vi "Read All Devices States.vi"(8 "error in (no error)":errorcluster, 11 "Data Cluster":T1 {"Flexi-Flow Devices"."Control State"."Control Mode" items=["Bus/RS232"=0, "FLOW-BUS slave"=2, "Valve close"=3, "Controller idle"=4, "Setpoint 100%"=7, "Valve fully open"=8, "Calibration mode"=9, "Setpoint 0%"=12, "RS232"=18, "Valve steering"=20, "Valve safe state"=22]}) -> (0 "error out":errorcluster, 1 "Array":sgl[](array[numeric]), 2 "Data Table":map{string, dbl}(c390), 3 "Array Out":T3[](array[typedef]) {"Control State"."Control Mode" items=["Bus/RS232"=0, "FLOW-BUS slave"=2, "Valve close"=3, "Controller idle"=4, "Setpoint 100%"=7, "Valve fully open"=8, "Calibration mode"=9, "Setpoint 0%"=12, "RS232"=18, "Valve steering"=20, "Valve safe state"=22]})   [LabVIEW 2024, in "FlexiFlowInterfaceCH2.lvlib"]
uses:
  FlexiFlowInterfaceCH2.lvlib
  Modbus Flexi-Flow State--cluster.ctl
  <vilib>/Plasmionique/MB Master/MB_Master_TCP/MB_Master_TCP.lvclass
  Device Type--enum.ctl
  Modbus Flexi-Flow Controls--cluster.ctl
  Modbus Flexi-Flow API/Control Mode--enum.ctl
  Modbus Flexi-Flow API/Control Function Values--enum.ctl
  Modbus Flexi-Flow Measure State--cluster.ctl
  Module Data--cluster.ctl
  Modbus TCP Connection Settings--cluster.ctl
  Modbus Flexi-Flow API/Bronkhorst Flexi-Flow ModbusTCP API.lvlib
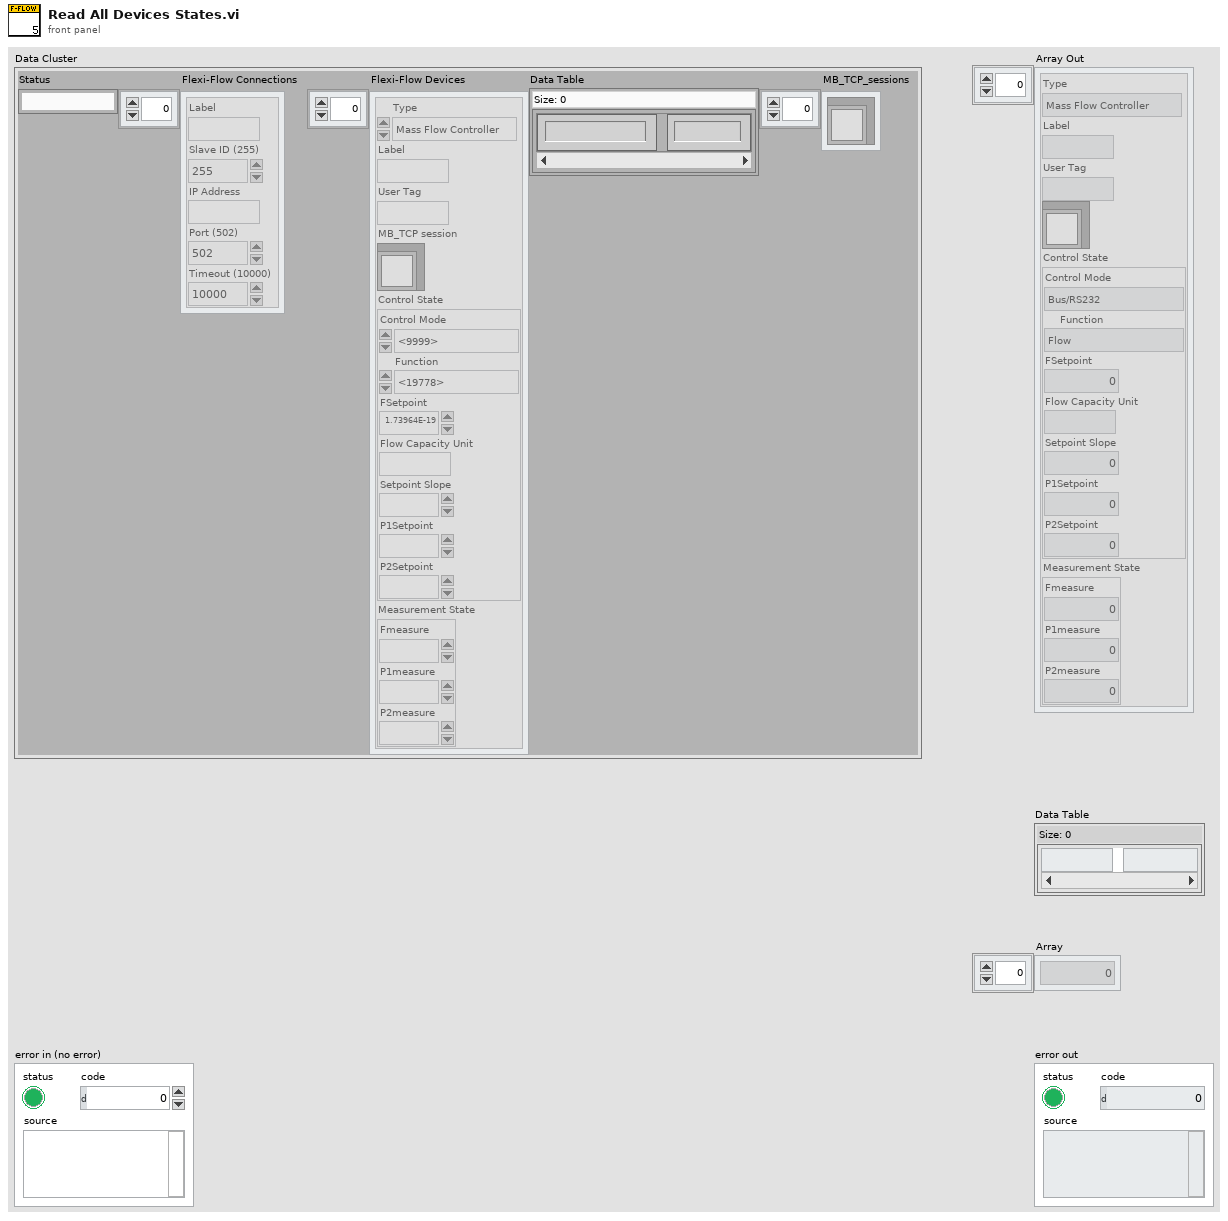
[diagram p1: front panel]
types:
  T1 = typedef "FlexiFlowInterfaceCH2.lvlib/Module Data--cluster.ctl" = cluster{"Status":string, "Flexi-Flow Connections":T2[], "Flexi-Flow Devices":T3[], "Data Table":map{string, dbl}, "MB_TCP_sessions":refnum<class "MB_Master_TCP.lvclass">[]}
  T2 = typedef "FlexiFlowInterfaceCH2.lvlib/Modbus TCP Connection Settings--cluster.ctl" = cluster{"Label":string, "Slave ID (255)":u8, "IP Address":string, "Port (502)":u16, "Timeout (10000)":i32}
  T3 = typedef "FlexiFlowInterfaceCH2.lvlib/Modbus Flexi-Flow State--cluster.ctl" = cluster{"Type":T4, "Label":string, "User Tag":string, "MB_TCP session":refnum<class "MB_Master_TCP.lvclass">, "Control State":T5, "Measurement State":T8}
  T4 = typedef "FlexiFlowInterfaceCH2.lvlib/Device Type--enum.ctl" = enum16{"Mass Flow Controller", "Mass Flow Meter"}
  T5 = typedef "FlexiFlowInterfaceCH2.lvlib/Modbus Flexi-Flow Controls--cluster.ctl" = cluster{"Control Mode":T6, "Function":T7, "FSetpoint":sgl, "Flow Capacity Unit":string, "Setpoint Slope":u16, "P1Setpoint":sgl, "P2Setpoint":sgl}
  T6 = typedef "Bronkhorst Flexi-Flow ModbusTCP API.lvlib/Control Mode--enum.ctl" = u16
  T7 = typedef "Bronkhorst Flexi-Flow ModbusTCP API.lvlib/Control Function Values--enum.ctl" = enum16{"Flow", "Upstream pressure", "Downstream pressure", "Flow with upstream pressure limit", "Flow with downstream pressure limit", "Upstream pressure with flow limit", "Downstream pressure with flow limit"}
  T8 = typedef "FlexiFlowInterfaceCH2.lvlib/Modbus Flexi-Flow Measure State--cluster.ctl" = cluster{"Fmeasure":dbl, "P1measure":sgl, "P2measure":sgl}
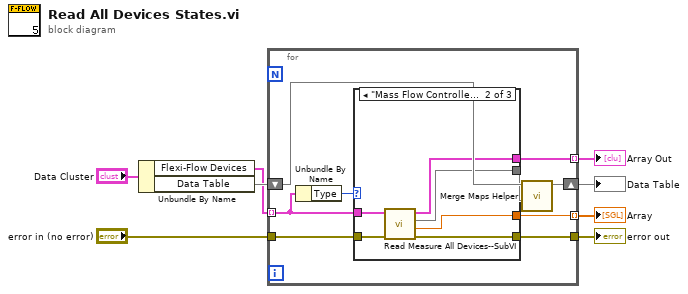
[diagram p0: block diagram]
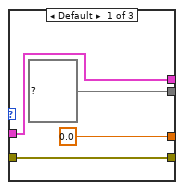
[diagram p2: hidden frame]
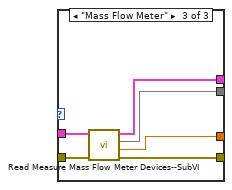
[diagram p3: hidden frame]
diagram:
  n1 = Unbundle By Name("Data Cluster") -> ("Flexi-Flow Devices"=w2:T3[], "Data Table"=w5:map{string, dbl})
  n2 = for {
    tunnel: w2 -> [w10] mode=indexing
    tunnel: [w15] -> w4 mode=indexing
    tunnel: "error in (no error)" -> [w17]
    tunnel: [w16] -> w8
    shift-right: [w13] -> w6
    shift-left: w5 -> [w14]
    tunnel: [w11] -> w7 mode=indexing
    n3 = Unbundle By Name(w10) -> ("Type"=w9:T4)
    n4 = case shown="\"Mass Flow Controller\"" w9 {
      tunnel: w17 -> [w19 w27 w32]
      tunnel: [w19 w26 w28] -> w16
      tunnel: [w21 w25 w31] -> w15
      tunnel: [map{string, dbl} {} ("map out") w24 w29] -> w12
      tunnel: [sgl 0.0 ("Value") w23 w30] -> w11
      tunnel: w10 -> [w21 w22 w33]
      frame Default {
      }
      frame "Mass Flow Controller" {
        n5 = call "Read Measure All Devices--SubVI.vi"("error in (no error)"=w27, "Flexi-Flow in"=w22) -> ("error out"=w26:errorcluster, "Value"=w23:sgl, "map out"=w24:map{string, dbl}, "Flexi-Flow out"=w25:T3)  [unwired: 6 in]
      }
      frame "Mass Flow Meter" {
        n6 = call "Read Measure Mass Flow Meter Devices--SubVI.vi"("error in (no error)"=w32, "Flexi-Flow in"=w33) -> ("error out"=w28:errorcluster, "Value"=w30:sgl, "map out"=w29:map{string, dbl}, "Flexi-Flow out"=w31:T3)  [unwired: 6 in]
      }
    }
    n7 = call "Merge Maps Helper.vi"("map in"=w12, "Data Table in"=w14) -> ("Data Table out"=w13:map{string, dbl})  [unwired: 9 in]
  }
  "error out" <- w8
  "Array" <- w7
  "Data Table" <- w6
  "Array Out" <- w4
